vi "Read Results from processing.vi"(8 "error in":errorcluster, 11 "CentralErrorHandlerDev runtime in":refnum<class "CentralErrorHandler runtime.lvclass">) -> (0 "error out":errorcluster, 2 "Results from processing":T1, 3 "CentralErrorHandlerDev runtime out":refnum<class "CentralErrorHandler runtime.lvclass">)   [LabVIEW 2014, in "CentralErrorHandler runtime.lvclass"]
uses:
  CentralErrorHandler runtime.lvclass
  configuration/result data indices.ctl
  CentralErrorHandler runtime.lvclass/CentralErrorHandler runtime.ctl
  configuration/CentralErrorHandler configuration.lvclass
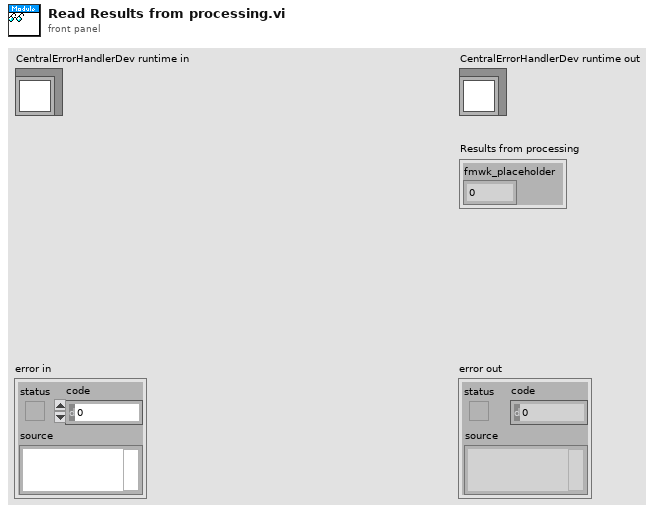
[diagram p1: front panel]
types:
  T1 = typedef "CentralErrorHandler configuration.lvclass/result data indices.ctl" = cluster{"fmwk_placeholder":i32}
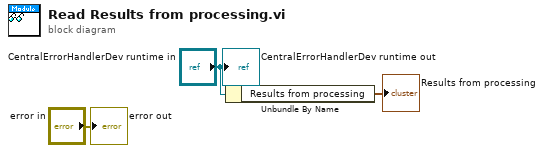
[diagram p0: block diagram]
diagram:
  n1 = Unbundle By Name("CentralErrorHandlerDev runtime in") -> ("Results from processing"=→"Results from processing":T1)
  "error out" <- "error in"
  "CentralErrorHandlerDev runtime out" <- "CentralErrorHandlerDev runtime in"
